vi "System_Initialize.vi"() -> (2 "TagBus DVR":refnum<data-value>, 3 "System DVR out":refnum<data-value>)   [LabVIEW 2015, in "System.lvclass"]
uses:
  System.lvclass
  TagBus/TagBus.lvclass
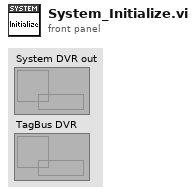
[diagram p1: front panel]
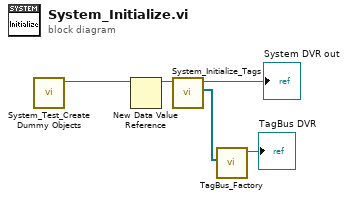
[diagram p0: block diagram]
diagram:
  n1 = call "System_Test_Create Dummy Objects.vi"() -> ("System.lvclass"=w4:refnum<class "System.lvclass">)  [unwired: 11 in]
  n2 = New Data Value Reference(data value=w4) -> (data value reference=w3:refnum<data-value>)  [unwired: 1 in, 1 out]
  n3 = call "System_Initialize_Tags.vi"("System DVR"=w3) -> ("TagDescriptions"=w5:refnum<class "tag descriptor.lvclass">[], "System DVR out"=→"System DVR out":refnum<data-value>)  [unwired: 9 in]
  n4 = call "TagBus_Factory.vi"("TagDescriptions"=w5) -> ("TagBus DVR"=→"TagBus DVR":refnum<data-value>)  [unwired: 10 in]
